vi "[Template] - Simple State Machine Module.vi"() -> ()   [LabVIEW 2015]
uses:
  TypeDefs/ENUM_State Template.ctl
  Utility/Universal Utility/FP/FPClass/(FP)/DecFrame_FP/DecFrame_FP.lvclass
  Utility/Universal Utility/TypeDefs_Utility/ENUM RB_Pos_Quadrant Position.ctl
  <vilib>/Utility/error.llb/DialogType.ctl
panel:
  in  "stop":bool
  out "Version":string
  out "State":T1=enum."Idle" caption="State ENUM (REPLACE)"
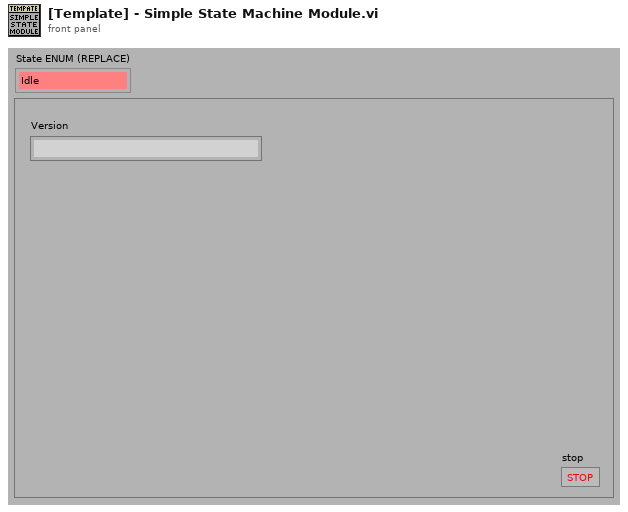
[diagram p1: front panel]
types:
  T1 = typedef "ENUM_State Template.ctl" = enum16{"<Startup>", "Idle", "STATE 1", "<Shutdown>"}
  T2 = enum32{"Invalid", "Standard", "Closed", "Hidden", "Minimized", "Maximized"}
  T3 = enum32{"invalid app kind", "Development System", "Run Time System", "Student Edition", "Embedded LabVIEW", "Evaluation", "Custom"}
  T4 = cluster{"App Kind":enum32{"invalid app kind", "Development System", "Run Time System", "Student Edition", "Embedded LabVIEW", "Evaluation", "Custom"}, "This VI":refnum<vi>, "Timeout":i32, "Module Name":string, "State":T1, "FP Data":refnum<class "DecFrame_FP.lvclass">, "FP State":enum32{"Invalid", "Standard", "Closed", "Hidden", "Minimized", "Maximized"}}
  T5 = typedef "ENUM RB_Pos_Quadrant Position.ctl" = enum32{"LFT-TOP", "MID-TOP", "RGT-TOP", "LFT-CTR", "MID-CTR", "RGT-CTR", "LFT-BOT", "MID-BOT", "RGT-BOT"}
  T6 = typedef "DialogType.ctl" = u16
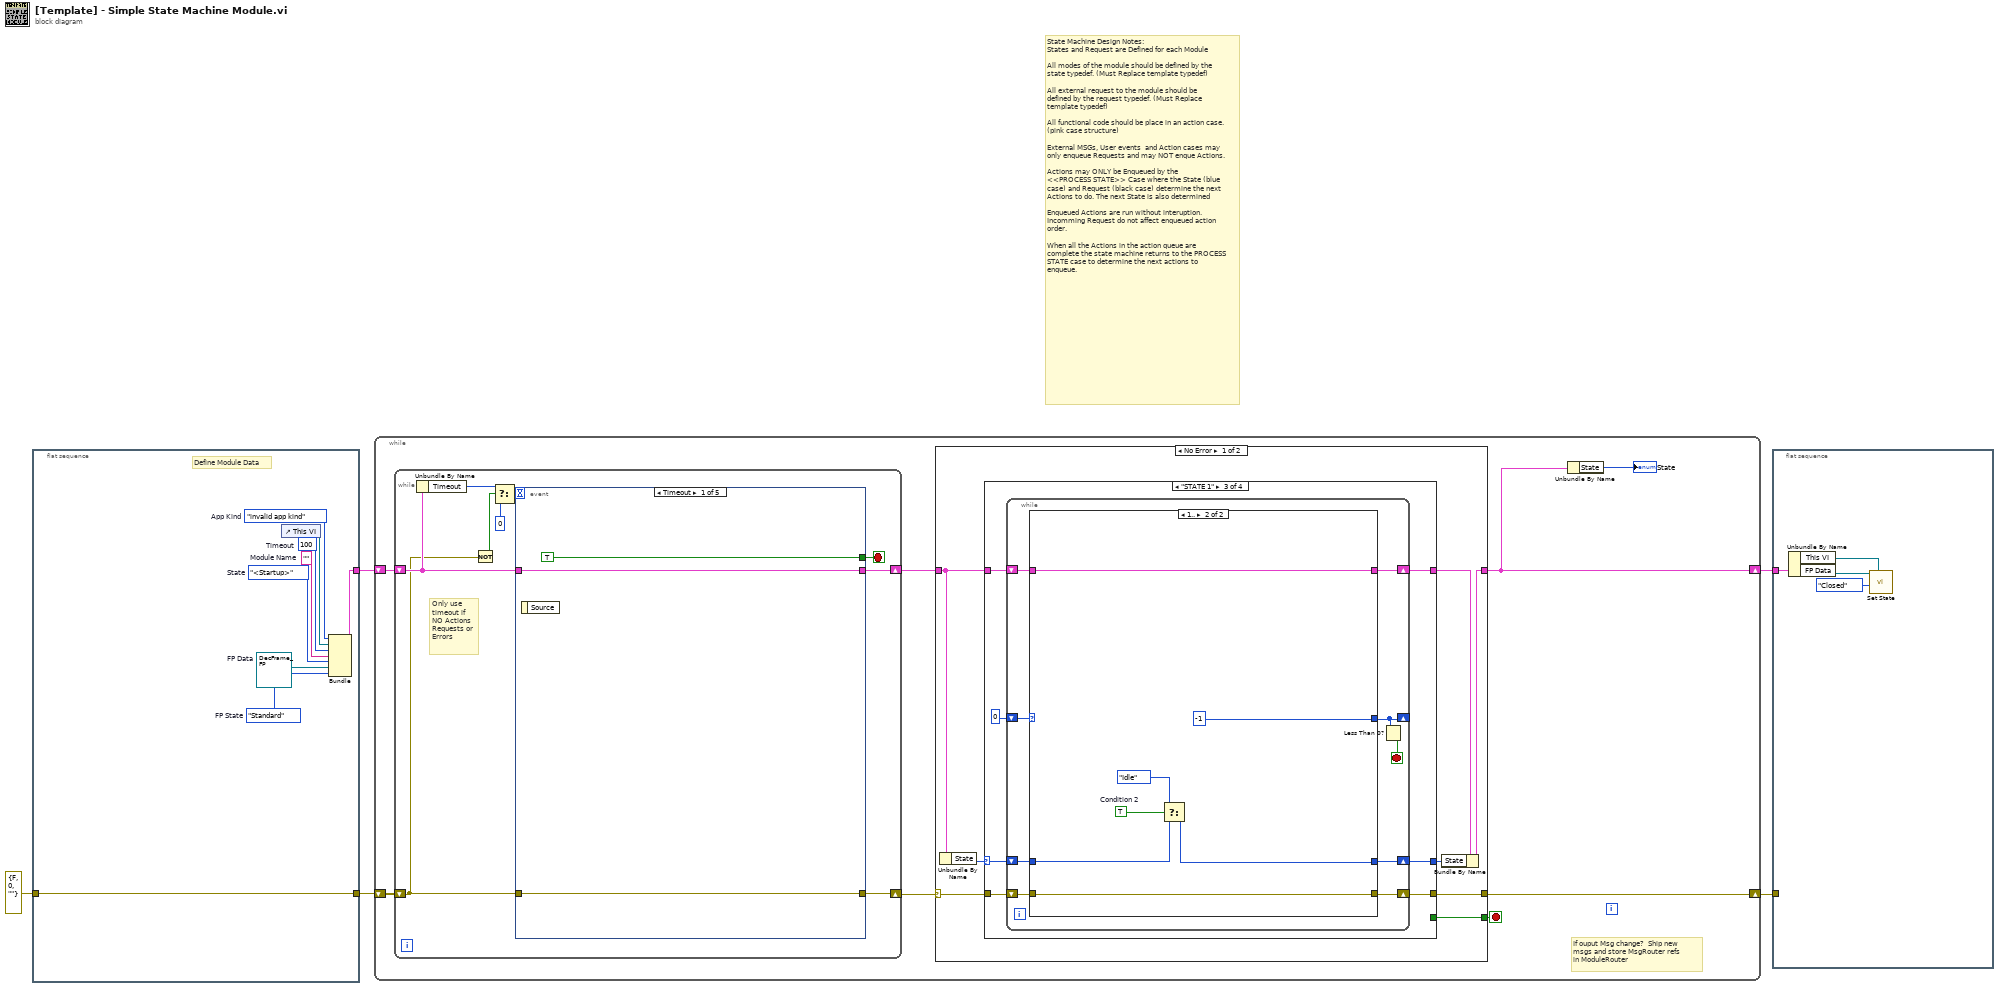
[diagram p0: block diagram]
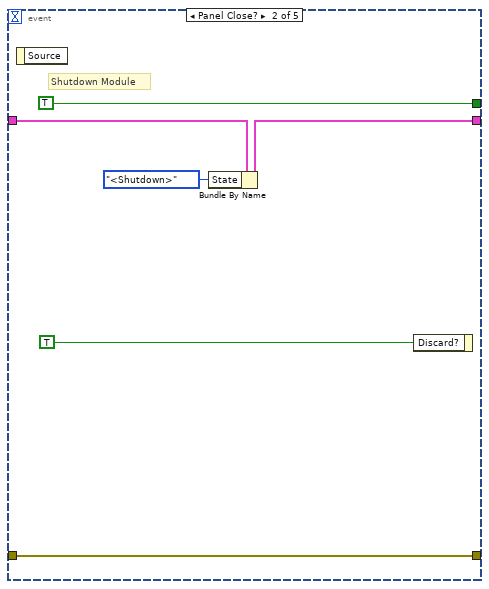
[diagram p2: hidden frame]
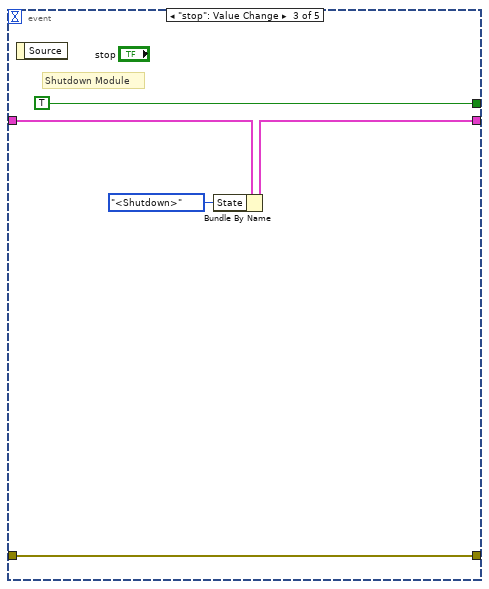
[diagram p3: hidden frame]
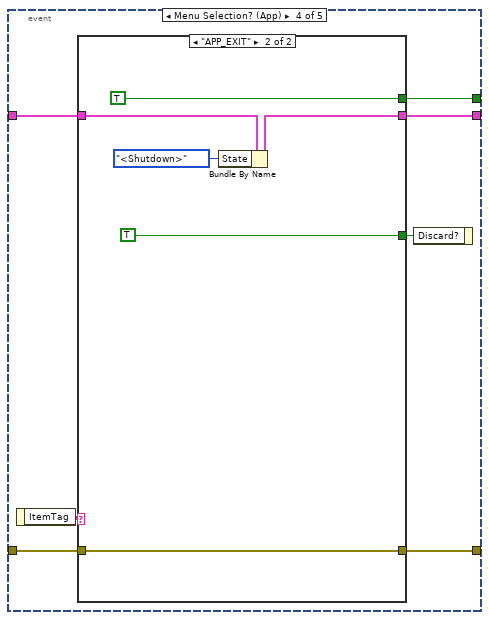
[diagram p4: hidden frame]
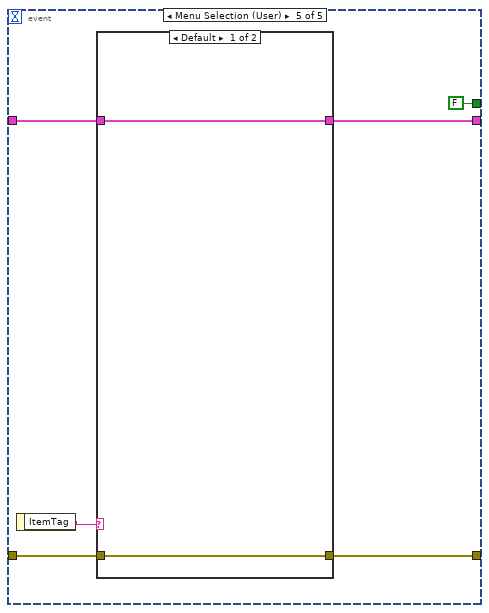
[diagram p6: hidden frame]
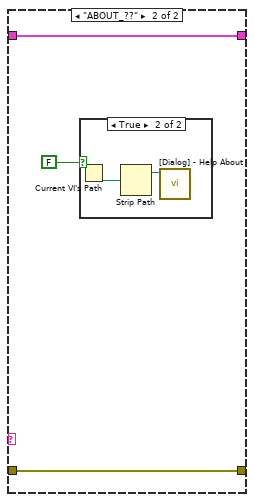
[diagram p7: hidden frame]
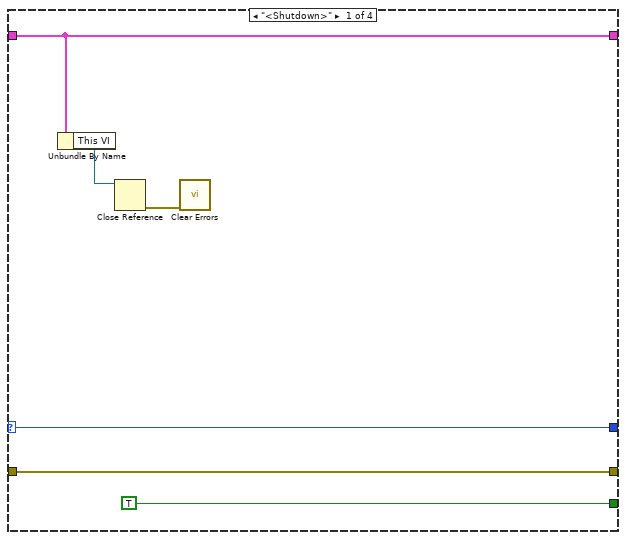
[diagram p9: hidden frame]
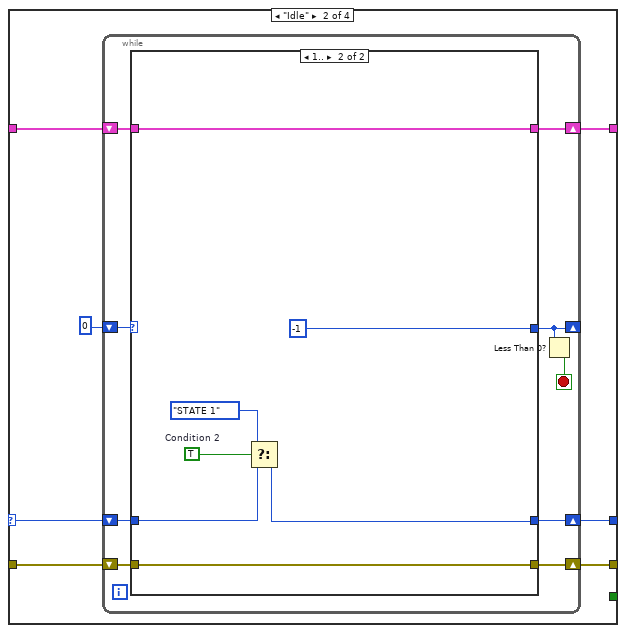
[diagram p10: hidden frame]
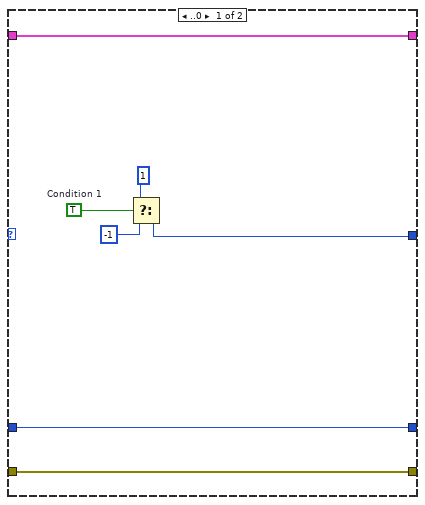
[diagram p11: hidden frame]
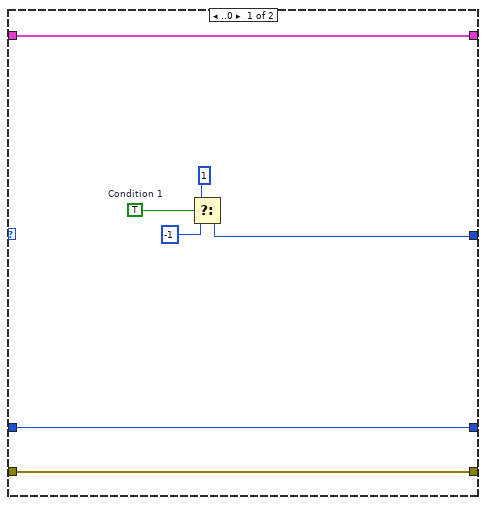
[diagram p12: hidden frame]
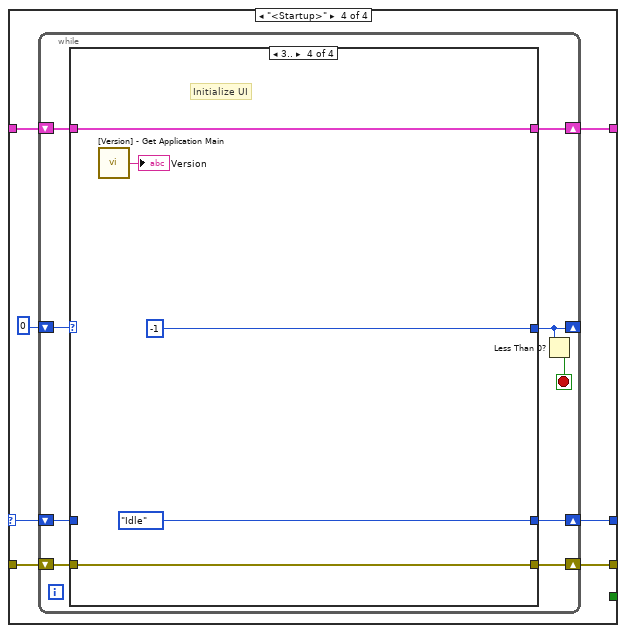
[diagram p13: hidden frame]
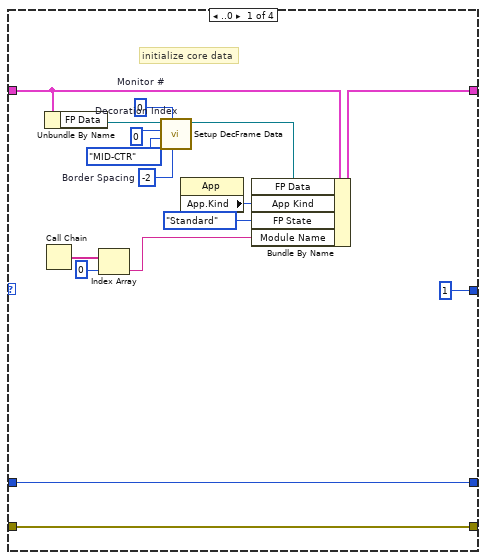
[diagram p14: hidden frame]
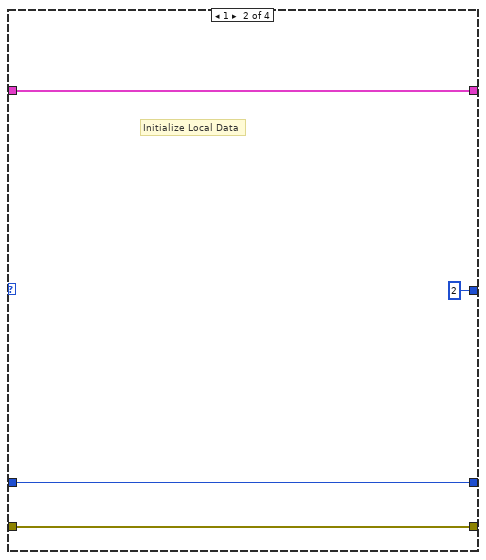
[diagram p15: hidden frame]
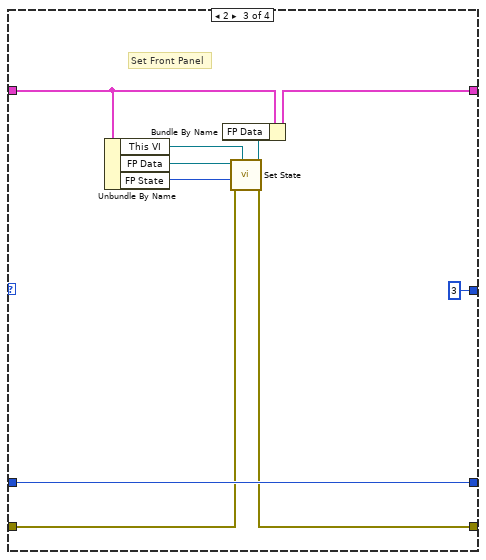
[diagram p16: hidden frame]
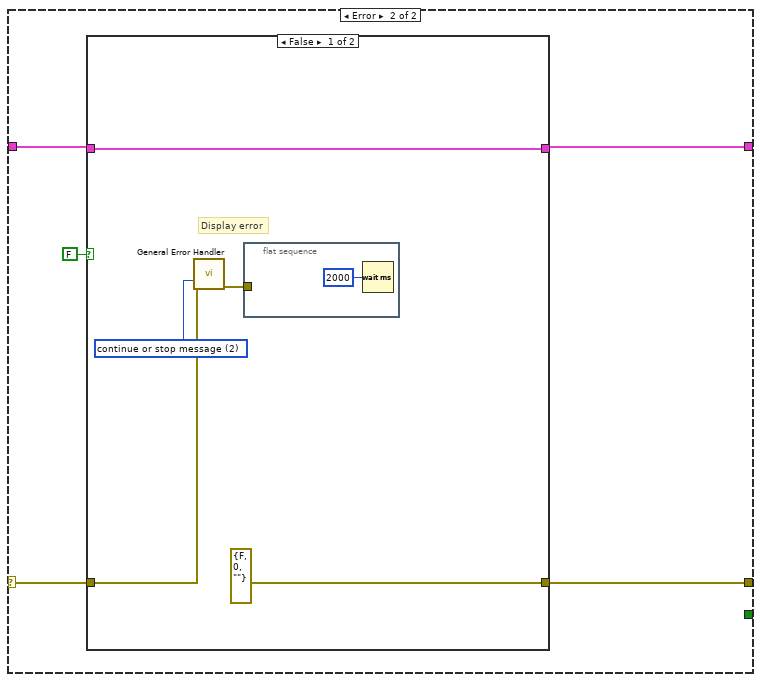
[diagram p17: hidden frame]
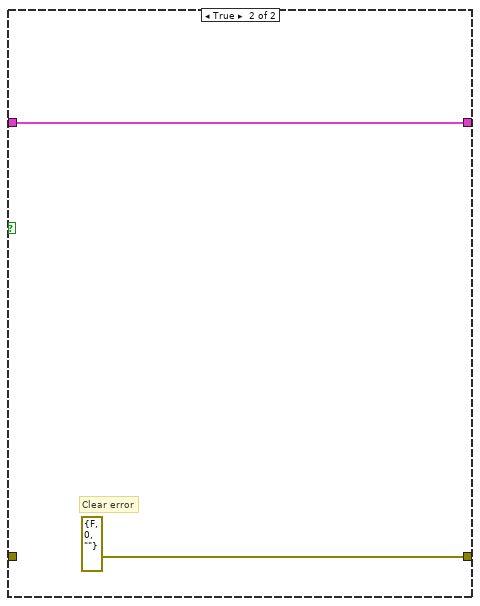
[diagram p18: hidden frame]
diagram:
  # "State Machine Design Notes:\nStates and Request are Defined for each Module\n\nAll modes of the module should be defined by the state typedef. (Must Replace template typedef)\n\nAll external request to the module should be\ndefined by the request typedef. (Must Replace template typedef)\n\nAll functional code should be place in an action case. (pink case structure)\n\nExternal MSGs, User events  and Action cases may only enqueue Requests and may NOT enque Actions.\n\nActions may ONLY be Enqueued by the\n<<PROCESS STATE>> Case where the State (blue case) and Request (black case) determine the next Actions to do. The next State is also determined\n\nEnqueued Actions are run without interuption.\nIncomming Request do not affect enqueued action order.\n\nWhen all the Actions in the action queue are complete the state machine returns to the PROCESS STATE case to determine the next actions to enqueue."
  n1 = flat-sequence {
    tunnel: errorcluster {"status"=FALSE, "code"=0, "source"=""} ("Error") -> [w14]
    tunnel: [w14] -> w4
    tunnel: [w13] -> w3
    frame #0 {
      w6 = T2."Standard"  # FP State
      w7 = refnum<class "DecFrame_FP.lvclass"> refnum  # FP Data
      w9 = ENUM_State_Template."<Startup>"  # State
      w11 = T3."invalid app kind"  # App Kind
      w12 = 100  # Timeout
      w8 = ""  # Module Name
      # "Define Module Data"
      n2 = control-ref of="This VI"() -> (w10:refnum<vi>)
      n3 = Bundle("App Kind"=w11, "This VI"=w10, "Timeout"=w12, "Module Name"=w8, "State"=w9, "FP Data"=w7, "FP State"=w6) -> (w13:T4)  [unwired: 1 in]
    }
  }
  n4 = while "JKI - String-Based Queued State Machine (Basic) v1.0" {
    shift-right: [w16] -> w2
    shift-left: w3 -> [w21]
    shift-right: [w15] -> w1
    shift-left: w4 -> [w20]
    stop <- w22 stop-if-true
    # "If ouput Msg change?  Ship new \nmsgs and store MsgRouter refs\nin ModuleRouter"
    n5 = while {
      shift-right: [w30] -> w17
      shift-left: w20 -> [w23]
      shift-right: [w31] -> w19
      shift-left: w21 -> [w24]
      stop <- w25 stop-if-true
      # "Only use\ntimeout if\nNO Actions\nRequests or\nErrors"
      n6 = Unbundle By Name(w24) -> ("Timeout"=w26:i32)
      n7 = Not(x=w23) -> (.not. x?=w29:bool)
      n8 = Select(t=w26, s=w29, f=0) -> (s? t:f=w27:i32)
      n9 = event shown="[0] Timeout" {
        selector: _ -> [_ _ _ _ _]
        dyn-events: _ -> [_ _ _ _ _]
        timeout: w27 -> [_ _ _ _ _]
        tunnel: w24 -> [w33 w37 w42 w49 w63]
        tunnel: [w34 w40 w45 w51 w65] -> w30
        tunnel: w23 -> [w34 w40 w45 w52 w66]
        tunnel: [w33 w36 w41 w48 w62] -> w31
        tunnel: [TRUE TRUE TRUE w46 FALSE] -> w25
        event Timeout {
          n10 = event-data() -> ()  [unwired: 1 in, 1 out]
        }
        event Panel Close? {
          # "Shutdown Module"
          n11 = event-data() -> ()  [unwired: 1 in, 1 out]
          n12 = Bundle By Name(cluster=w37, "State"=ENUM_State_Template."<Shutdown>") -> (w36:T4)
          n13 = event-data("Discard?"=TRUE) -> ()  [unwired: 1 in, 1 out]
        }
        event "stop": Value Change {
          # "Shutdown Module"
          n14 = event-data() -> ()  [unwired: 1 in, 1 out]
          n15 = Bundle By Name(cluster=w42, "State"=ENUM_State_Template."<Shutdown>") -> (w41:T4)
        }
        event Menu Selection? (App) {
          n16 = event-data() -> ("ItemTag"=w50:string)  [unwired: 1 in]
          n17 = case shown="\"APP_EXIT\"" w50 {
            tunnel: [w54 w60] -> w51
            tunnel: w52 -> [w54 w60]
            tunnel: [_ TRUE] -> w47
            tunnel: w49 -> [w53 w57]
            tunnel: [w53 w56] -> w48
            tunnel: [_ TRUE] -> w46
            frame Default {
            }
            frame "APP_EXIT" {
              n18 = Bundle By Name(cluster=w57, "State"=ENUM_State_Template."<Shutdown>") -> (w56:T4)
            }
          }
          n19 = event-data("Discard?"=w47) -> ()  [unwired: 1 in, 1 out]
        }
        event Menu Selection (User) {
          n20 = event-data() -> ("ItemTag"=w64:string)  [unwired: 1 in]
          n21 = case shown="Default" w64 {
            tunnel: [w68 w71] -> w65
            tunnel: w66 -> [w68 w71]
            tunnel: w63 -> [w67 w70]
            tunnel: [w67 w70] -> w62
            frame Default {
            }
            frame "ABOUT_??" {
              n22 = case shown="True" FALSE {
                frame False {
                }
                frame True {
                  n23 = Current VI's Path() -> (path=w73:path)
                  n24 = Strip Path(path=w73) -> (stripped path=w72:path)  [unwired: 1 out]
                  n25 = call "[Dialog] - Help About.vi"("Path"=w72) -> ()  [unwired: 11 in]
                }
              }
            }
          }
        }
      }
    }
    n26 = case shown="No Error" w17 {
      selector: w17 -> [w74 w199]
      tunnel: w19 -> [w81 w202]
      tunnel: [w79 w200] -> w15
      tunnel: [w75 _] -> w22
      tunnel: [w77 w201] -> w16
      frame No Error {
        n27 = Unbundle By Name(w81) -> ("State"=w80:T1)
        n28 = case shown="\"STATE 1\"" w80 {
          selector: w80 -> [w83 w93 w123 w153]
          tunnel: [w82 w88 w118 w150] -> w79
          tunnel: w81 -> [w85 w94 w124 w154]
          tunnel: [w85 w91 w121 w151] -> w78
          tunnel: [w83 w90 w120 w149] -> w76
          tunnel: [TRUE _ _ _] -> w75
          tunnel: w74 -> [w82 w89 w119 w148]
          frame "<Shutdown>" {
            n29 = Unbundle By Name(w85) -> ("This VI"=w86:refnum<vi>)
            n30 = Close Reference(reference=w86) -> (error out=w87:errorcluster)  [unwired: 1 in]
            n31 = call <vilib>:"Clear Errors.vi"("error in (no error)"=w87) -> ()  [unwired: 5 in, 2 out]
          }
          frame "Idle" {
            n32 = while {
              shift-right: [w99] -> w90
              shift-left: w93 -> [w100]
              shift-right: [w97] -> w91
              shift-left: w94 -> [w98]
              shift-right: [w101] -> _
              shift-left: 0 -> [w103]
              shift-right: [w95] -> w88
              shift-left: w89 -> [w96]
              stop <- w102 stop-if-true
              n33 = case shown="1.." w103 {
                tunnel: [w107 -1 ("t")] -> w101
                tunnel: w100 -> [w105 w114]
                tunnel: [w105 w113] -> w99
                tunnel: w98 -> [w110 w117]
                tunnel: [w110 w117] -> w97
                tunnel: w96 -> [w104 w111]
                tunnel: [w104 w111] -> w95
                frame ..0 {
                  w106 = TRUE  # Condition 1
                  n34 = Select(t=1, s=w106, f=-1) -> (s? t:f=w107:i32)
                }
                frame 1.. {
                  w116 = TRUE  # Condition 2
                  n35 = Select(t=ENUM_State_Template."STATE 1", s=w116, f=w114) -> (s? t:f=w113:T1)
                }
              }
              n36 = Less Than 0?(x=w101) -> (x < 0?=w102:bool)
            }
          }
          frame "STATE 1" {
            n37 = while {
              shift-right: [w127] -> w118
              shift-left: w119 -> [w128]
              shift-right: [w129] -> w120
              shift-left: w123 -> [w130]
              shift-right: [w125] -> w121
              shift-left: w124 -> [w126]
              shift-right: [w131] -> _
              shift-left: 0 -> [w133]
              stop <- w132 stop-if-true
              n38 = case shown="1.." w133 {
                tunnel: [w136 -1 ("t")] -> w131
                tunnel: w130 -> [w134 w143]
                tunnel: [w134 w142] -> w129
                tunnel: w128 -> [w140 w147]
                tunnel: [w140 w147] -> w127
                tunnel: w126 -> [w139 w146]
                tunnel: [w139 w146] -> w125
                frame ..0 {
                  w135 = TRUE  # Condition 1
                  n39 = Select(t=1, s=w135, f=-1) -> (s? t:f=w136:i32)
                }
                frame 1.. {
                  w145 = TRUE  # Condition 2
                  n40 = Select(t=ENUM_State_Template."Idle", s=w145, f=w143) -> (s? t:f=w142:T1)
                }
              }
              n41 = Less Than 0?(x=w131) -> (x < 0?=w132:bool)
            }
          }
          frame "<Startup>" {
            n42 = while {
              shift-right: [w157] -> w150
              shift-left: w148 -> [w158]
              shift-right: [w159] -> w149
              shift-left: w153 -> [w160]
              shift-right: [w155] -> w151
              shift-left: w154 -> [w156]
              shift-right: [w161] -> _
              shift-left: 0 -> [w163]
              stop <- w162 stop-if-true
              n43 = case shown="3.." w163 {
                tunnel: [1 ("t") 2 ("t") 3 ("t") -1 ("t")] -> w161
                tunnel: w160 -> [w179 w181 w193 _]
                tunnel: [w179 w181 w193 ENUM_State_Template."Idle" ("State")] -> w159
                tunnel: w158 -> [w164 w183 w188 w198]
                tunnel: [w164 w183 w187 w198] -> w157
                tunnel: w156 -> [w167 w182 w191 w197]
                tunnel: [w168 w182 w190 w197] -> w155
                frame ..0 {
                  w169 = i16 -2  # Border Spacing
                  w173 = 0  # Decoration Index
                  w174 = u16 0  # Monitor #
                  # "initialize core data"
                  n44 = Call Chain() -> (call chain=w177:string[])
                  n45 = Unbundle By Name(w167) -> ("FP Data"=w175:refnum<class "DecFrame_FP.lvclass">)
                  n46 = Index Array(array=w177, index=0) -> (element=w176:string)
                  n47 = call-dynamic "Setup DecFrame Data.vi"("Border Spacing"=w169, "Monitor #"=w174, "FPLocation"=ENUM_RB_Pos_Quadrant_Position."MID-CTR", "Decoration Index"=w173, "(FP)"=w175) -> ("(FP) Out"=w171:refnum<class "DecFrame_FP.lvclass">)  [unwired: 5 in, 1 out]
                  n48 = property class="App"() -> ("App.Kind"=w172:T3)  [unwired: 2 in, 2 out]
                  n49 = Bundle By Name(cluster=w167, "FP Data"=w171, "App Kind"=w172, "FP State"=T2."Standard" ("State"), "Module Name"=w176) -> (w168:T4)
                }
                frame 1 {
                  # "Initialize Local Data"
                }
                frame 2 {
                  # "Set Front Panel"
                  n50 = Unbundle By Name(w191) -> ("This VI"=w184:refnum<vi>, "FP Data"=w192:refnum<class "DecFrame_FP.lvclass">, "FP State"=w185:T2)
                  n51 = call-dynamic "Set State.vi"("VI Ref"=w184, "Error"=w188, "State"=w185, "(FP)"=w192) -> ("Error Out"=w187:errorcluster, "(FP) Out"=w189:refnum<class "DecFrame_FP.lvclass">)  [unwired: 5 in, 1 out]
                  n52 = Bundle By Name(cluster=w191, "FP Data"=w189) -> (w190:T4)
                }
                frame 3.. {
                  # "Initialize UI"
                  n53 = call "[Version] - Get Application Main.vi"() -> ("Version"=→"Version":string)
                }
              }
              n54 = Less Than 0?(x=w161) -> (x < 0?=w162:bool)
            }
          }
        }
        n55 = Bundle By Name(cluster=w78, "State"=w76) -> (w77:T4)
      }
      frame Error {
        n56 = case shown="False" FALSE {
          tunnel: w199 -> [w208 _]
          tunnel: [w207 w210] -> w201
          tunnel: w202 -> [w207 w210]
          tunnel: [errorcluster {"status"=FALSE, "code"=0, "source"=""} ("error out") errorcluster {"status"=FALSE, "code"=0, "source"=""} ("error out")] -> w200
          frame False {
            w204 = T6 2 items=["no dialog", "OK message", "continue or stop message", "OK message + warnings", "continue/stop + warnings"] ("type of dialog (OK msg:1)")
            # "Display error"
            n57 = call <vilib>:"General Error Handler.vi"("type of dialog (OK msg:1)"=w204, "error in (no error)"=w208) -> ("error out"=w205:errorcluster)  [unwired: 9 in, 4 out]
            n58 = flat-sequence {
              tunnel: w205 -> [_]
              frame #0 {
                n59 = Wait (ms)(milliseconds to wait=u32 2000) -> ()  [unwired: 1 out]
              }
            }
          }
          frame True {
            # "Clear error"
          }
        }
      }
    }
    n60 = Unbundle By Name(w16) -> ("State"=→"State":T1)
  }
  n61 = flat-sequence {
    tunnel: w2 -> [w215]
    tunnel: w1 -> [_]
    frame #0 {
      n62 = Unbundle By Name(w215) -> ("This VI"=w213:refnum<vi>, "FP Data"=w214:refnum<class "DecFrame_FP.lvclass">)
      n63 = call-dynamic "Set State.vi"("VI Ref"=w213, "State"=T2."Closed", "(FP)"=w214) -> ()  [unwired: 6 in, 3 out]
    }
  }
